vi "scanStatusView.vi"(10 "UserEvents in":refnum<class "UserEvents.lvclass">) -> ()   [LabVIEW 2015, in "FAMTViews.lvlib"]
uses:
  FAMTViews.lvlib
  UserEvents/UserEvents.lvclass
  UserEvents/UserEvents.lvclass/UserEvents.ctl
  Typedefs/StateSelector.ctl
  Typedefs/FAMTTypedefs.lvlib
panel:
  out "Current Amplitude":dbl format="%.3f"
  out "Current Rate":string
  out "Current Demand":dbl[unit] format="%.3f"
  out "Amplitude Total":u16
  out "Amplitude Step":u16
  out "Rate Total":u16
  out "Rate Step":u16
  out "Waveform Total":u16
  out "Waveform Step":u16
  # "of"
  # "Hz"
  # "of"
  # "of"
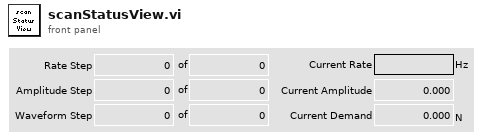
[diagram p1: front panel]
types:
  T1 = typedef "FAMTTypedefs.lvlib/PubDataEvents.ctl" = cluster{"State":refnum<user-event>, "ErrorCode":refnum<user-event>, "ADC Outputs":refnum<user-event>, "InputData":refnum<user-event>, "ControllerData":refnum<user-event>, "TestStatus":refnum<user-event>, "LogPath":refnum<user-event>, "ILC Outputs":refnum<user-event>, "Scan Progress":refnum<user-event>}
  T2 = cluster{"Event Registration Refnum":refnum<event-registration>, "Event Registration Refnum":refnum<event-registration>}
  T3 = typedef "FAMTTypedefs.lvlib/StateSelector.ctl" = enum16{"OfflineState", "FaultState", "StandbyState", "DisabledState", "EnabledState", "WaitForUserInputState", "PerformOpenLoopScanState"}
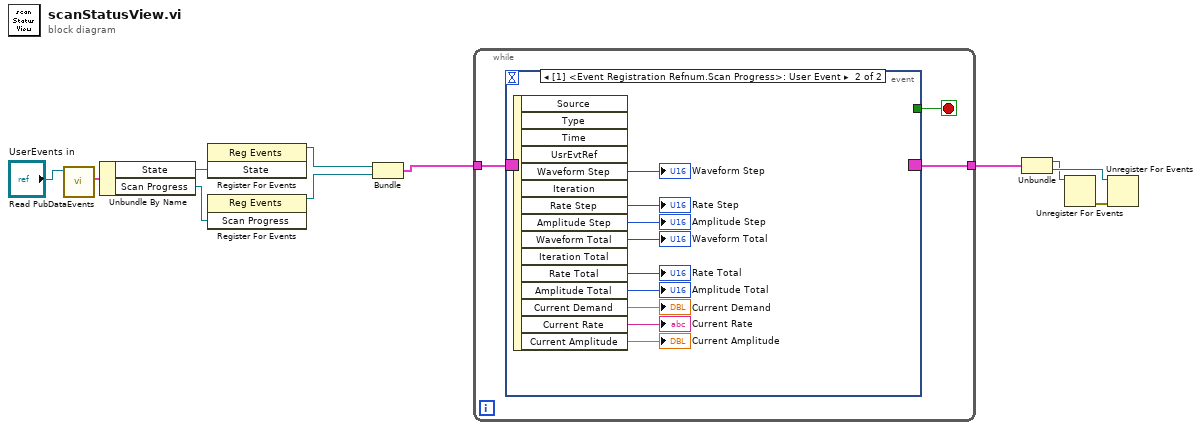
[diagram p0: block diagram]
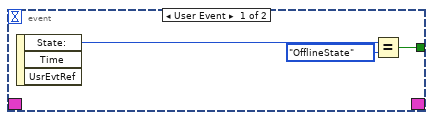
[diagram p2: hidden frame]
diagram:
  n1 = call "Read PubDataEvents.vi"("UserEvents in"="UserEvents in") -> ("PubDataEvents"=w10:T1)  [unwired: 9 in, 1 out]
  n2 = Unbundle By Name(w10) -> ("State"=w9:refnum<user-event>, "Scan Progress"=w11:refnum<user-event>)
  n3 = register-events(w9) -> (reference out=w4:refnum<event-registration>)  [unwired: 2 in, 1 out]
  n4 = register-events(w11) -> (reference out=w5:refnum<event-registration>)  [unwired: 2 in, 1 out]
  n5 = Bundle("Event Registration Refnum"=w4, "Event Registration Refnum"=w5) -> (w3:T2)  [unwired: 1 in]
  n6 = while {
    tunnel: w3 -> [w14]
    tunnel: [w13] -> w2
    stop <- w12 stop-if-true
    n7 = event shown="[1] <Event Registration Refnum.Scan Progress>: User Event" {
      selector: w14 -> [_ _]
      dyn-events: [_ _] -> w13
      timeout: _ -> [_ _]
      tunnel: [w16 _] -> w12
      event User Event {
        n8 = event-data() -> ("State:"=w15:T3)  [unwired: 1 in, 2 out]
        n9 = Equal?(x=w15, y=StateSelector."OfflineState") -> (x = y?=w16:bool)
      }
      event User Event {
        n10 = event-data() -> ("Waveform Step"=→"Waveform Step":u16, "Rate Step"=→"Rate Step":u16, "Amplitude Step"=→"Amplitude Step":u16, "Waveform Total"=→"Waveform Total":u16, "Rate Total"=→"Rate Total":u16, "Amplitude Total"=→"Amplitude Total":u16, "Current Demand"=→"Current Demand":dbl[unit], "Current Rate"=→"Current Rate":string, "Current Amplitude"=→"Current Amplitude":dbl)  [unwired: 1 in, 6 out]
      }
    }
  }
  n11 = Unbundle(w2) -> ("Event Registration Refnum"=w1:refnum<event-registration>, "Event Registration Refnum"=w6:refnum<event-registration>)
  n12 = Unregister For Events(event registration refnum=w1) -> (error out=w7:errorcluster)  [unwired: 1 in]
  n13 = Unregister For Events(event registration refnum=w6, error in=w7) -> ()  [unwired: 1 out]
